vi "Save File DOE Model Number and Folder Setup.vi"(9 "LV Program":T1=enum."DOE Stand", 10 "Network Model Location":path, 11 "All Models Excel Sheet":path) -> (2 "Header":string[](array[string]), 3 "Model Data":string[][](array[string]))   [LabVIEW 2016, in "File Setup.lvlib"]
doc: "This VI will create a Archive folder and check to see if there \nis a newer version of the \"Model Information\" excel worksheet.\nIf there is a newer version, it will move the older version to the\nArchive folder, copy the new version to the local machine, and open\nthe excel file and save it as a .csv. This will improve performance the next\ntime the program is run.\n\nIf there is no new version, it will open the .csv file (created above)."
uses:
  File Setup.lvlib
  File Setup (Public)/Type Definition/Save File DOE LabView Program.ctl
panel:
  out "Latest File on Network Folder":path
  out "error out":errorcluster
  in  "error in (no error)":errorcluster
  # "This VI will create a Archive folder and check to see if there \nis a newer version of the \"Model Information\" excel worksheet.\nIf there is a newer version, it will move the older version to the\nArchive folder, copy the new version to the local machine, and open\nthe excel file and save it as a .csv. This will improve performance the next\ntime the program is run.\n\nIf there is no new version, it will open the .csv file (created above)."
  # "Header File to allow for searching elsewhere in the program"
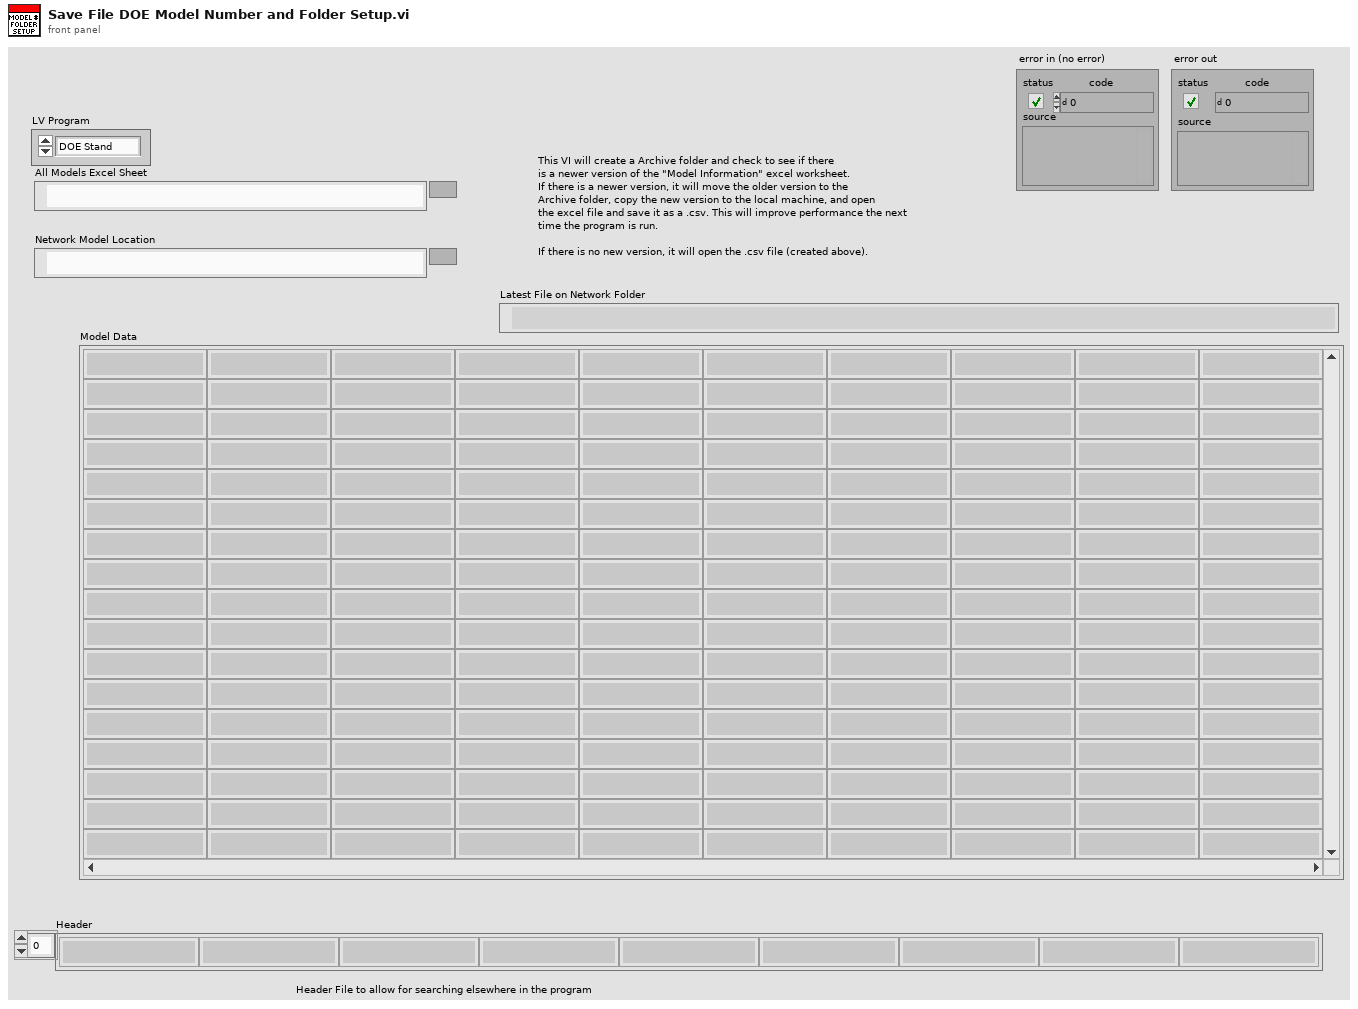
[diagram p1: front panel]
types:
  T1 = typedef "File Setup.lvlib/Save File DOE LabView Program.ctl" = enum16{"No Name Found", "DOE Stand", "Dishwasher Kitchen", "Portable Stand", "HEWH", "Dryer", "Dryer WILT", "HCC", "PRAT", "HEWH RLT"}
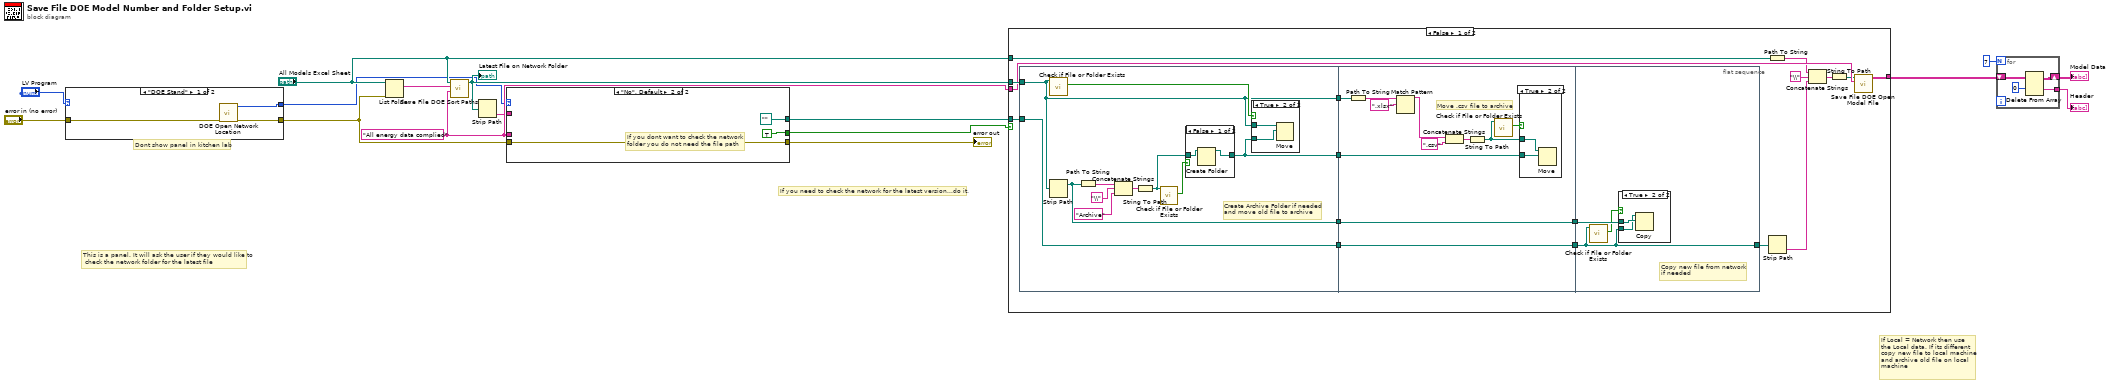
[diagram p0: block diagram]
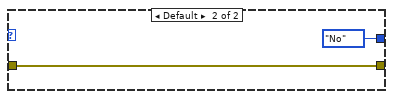
[diagram p2: hidden frame]
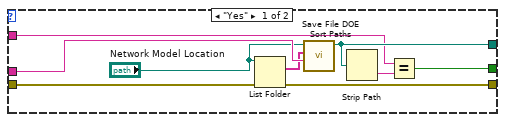
[diagram p3: hidden frame]
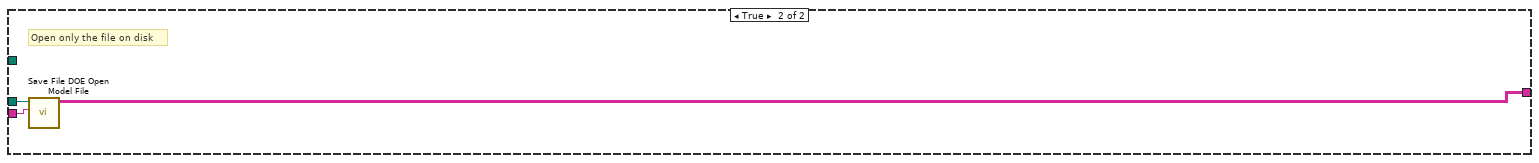
[diagram p8: hidden frame]
diagram:
  w14 = "All energy data complied" ("regular expression")
  # "Dont show panel in kitchen lab"
  # "This is a panel. It will ask the user if they would like to\n check the network folder for the latest file"
  # "If you need to check the network for the latest version...do it."
  # "If Local = Network then use \nthe Local data. If its different \ncopy new file to local machine\nand archive old file on local\nmachine"
  n1 = case shown="\"DOE Stand\"" "LV Program" {
    tunnel: [w19 enum16{"", "No", "Yes"}."No" ("Check Folder Output")] -> w4
    tunnel: [w18 w20] -> w3
    tunnel: "error in (no error)" -> [w17 w20]
    frame "DOE Stand" {
      n2 = call "DOE Open Network Location.vi"("error in (no error)"=w17) -> ("error out"=w18:errorcluster, "Check Folder Output"=w19:enum16{"", "No", "Yes"})  [unwired: 9 in]
    }
    frame Default {
    }
  }
  n3 = List Folder(path="All Models Excel Sheet", error in=w3) -> (filenames=w13:string[])  [unwired: 2 in, 3 out]
  n4 = call "Save File DOE Sort Paths.vi"("Search Expression"=w14, "filenames"=w13, "Folder Path"="All Models Excel Sheet") -> ("Latest File on Network Folder"=w15:path)  [unwired: 7 in, 1 out]
  "Latest File on Network Folder" <- w15
  n5 = Strip Path(path=w15) -> (name=w11:string)  [unwired: 1 out]
  n6 = case shown="\"No\", Default" w4 {
    tunnel: w14 -> [w30 _]
    tunnel: [w29 path "" ("Latest File on Network Folder")] -> w12
    tunnel: w11 -> [w27 _]
    tunnel: [w24 TRUE] -> w6
    tunnel: w3 -> [w23 w31]
    tunnel: [w22 w31] -> w1
    frame "Yes" {
      n7 = List Folder(path="Network Model Location", error in=w23) -> (filenames=w25:string[], error out=w22:errorcluster)  [unwired: 2 in, 2 out]
      n8 = call "Save File DOE Sort Paths.vi"("Search Expression"=w30, "filenames"=w25, "Folder Path"="Network Model Location") -> ("Latest File on Network Folder"=w29:path)  [unwired: 7 in, 1 out]
      n9 = Strip Path(path=w29) -> (name=w28:string)  [unwired: 1 out]
      n10 = Equal?(x=w27, y=w28) -> (x = y?=w24:bool)
    }
    frame "No", Default {
      # "If you dont want to check the network\nfolder you do not need the file path"
    }
  }
  "error out" <- w1
  n11 = case shown="False" w6 {
    tunnel: [w42 w87] -> w10
    tunnel: w15 -> [w50 w86]
    tunnel: w14 -> [w41 w85]
    tunnel: w12 -> [w46 _]
    tunnel: "All Models Excel Sheet" -> [w39 _]
    frame False {
      n12 = flat-sequence {
        tunnel: w50 -> [w54]
        tunnel: [w54] -> w49
        tunnel: [w53] -> w48
        tunnel: [w52] -> w47
        tunnel: w46 -> [w52]
        tunnel: [w51] -> w44
        tunnel: w49 -> [w71]
        tunnel: w48 -> [w70]
        tunnel: w47 -> [w69]
        tunnel: [w69] -> w45
        tunnel: w44 -> [w68]
        tunnel: [w68] -> w43
        tunnel: w45 -> [w80]
        tunnel: w43 -> [w82]
        tunnel: [w80] -> w40
        frame #0 {
          # "Create Archive Folder if needed\nand move old file to archive"
          n13 = call <vilib>:"Check if File or Folder Exists.vi"("path"=w54) -> ("file or folder exists?"=w55:bool)  [unwired: 8 in, 2 out]
          n14 = Strip Path(path=w54) -> (stripped path=w51:path)  [unwired: 1 out]
          n15 = Path To String(path=w51) -> (string=w56:string)
          n16 = Concatenate Strings(w56, "\\" ("string"), "Archive" ("Search Expression")) -> (w59:string)
          n17 = String To Path(string=w59) -> (path=w61:path)
          n18 = call <vilib>:"Check if File or Folder Exists.vi"("path"=w61) -> ("file or folder exists?"=w60:bool)  [unwired: 8 in, 2 out]
          n19 = case shown="False" w60 {
            tunnel: w61 -> [w65 w66]
            tunnel: [w64 w66] -> w53
            frame False {
              n20 = Create Folder(path (use dialog)=w65) -> (created path=w64:path)  [unwired: 2 in, 2 out]
            }
            frame True {
            }
          }
          n21 = case shown="True" w55 {
            tunnel: w53 -> [_ w63]
            tunnel: w54 -> [_ w62]
            frame False {
            }
            frame True {
              n22 = Move(source path=w62, 10:w63) -> ()  [unwired: 3 in, 3 out]
            }
          }
        }
        frame #1 {
          # "Move .csv file to archive"
          n23 = Path To String(path=w71) -> (string=w73:string)
          n24 = Match Pattern(string=w73, regular expression=".xlsx") -> (before substring=w75:string)  [unwired: 1 in, 3 out]
          n25 = Concatenate Strings(w75, ".csv" ("replace string (\"\")")) -> (w77:string)
          n26 = String To Path(string=w77) -> (path=w67:path)
          n27 = call <vilib>:"Check if File or Folder Exists.vi"("path"=w67) -> ("file or folder exists?"=w72:bool)  [unwired: 8 in, 2 out]
          n28 = case shown="True" w72 {
            tunnel: w70 -> [_ w79]
            tunnel: w67 -> [_ w78]
            frame False {
            }
            frame True {
              n29 = Move(source path=w78, 10:w79) -> ()  [unwired: 3 in, 3 out]
            }
          }
        }
        frame #2 {
          # "Copy new file from network\nif needed"
          n30 = call <vilib>:"Check if File or Folder Exists.vi"("path"=w80) -> ("file or folder exists?"=w81:bool)  [unwired: 8 in, 2 out]
          n31 = case shown="True" w81 {
            tunnel: w82 -> [_ w84]
            tunnel: w80 -> [_ w83]
            frame False {
            }
            frame True {
              n32 = Copy(10:w84, 11:w83) -> ()  [unwired: 3 in, 3 out]
            }
          }
        }
      }
      n33 = Path To String(path=w39) -> (string=w38:string)
      n34 = Strip Path(path=w40) -> (name=w36:string)  [unwired: 1 out]
      n35 = Concatenate Strings(w38, "\\" ("string"), w36) -> (w35:string)
      n36 = String To Path(string=w35) -> (path=w34:path)
      n37 = call "Save File DOE Open Model File.vi"("regular expression"=w41, "All Models Excel Sheet"=w34) -> ("all rows"=w42:string[][])  [unwired: 9 in]
    }
    frame True {
      # "Open only the file on disk"
      n38 = call "Save File DOE Open Model File.vi"("regular expression"=w85, "All Models Excel Sheet"=w86) -> ("all rows"=w87:string[][])  [unwired: 9 in]
    }
  }
  n39 = for {
    N: 7 -> [_]
    shift-right: [w89] -> w8
    shift-left: w10 -> [w91]
    tunnel: [w88] -> w7
    n40 = Delete From Array(array=w91, index (row)=0) -> (deleted portion=w88:string[], array with subset deleted=w89:string[][])  [unwired: 2 in]
  }
  "Model Data" <- w8
  "Header" <- w7
